vi "Validate Timing.vi"(8 "error in (no error)":errorcluster, 10 "Mode":T3="Standard-mode", 11 "I2C timing (ns)":T1 {"fSCL" format="%#_6p"}) -> (0 "error out":errorcluster, 1 "Timing violations":T2, 2 "Timing passed?":bool, 3 "I2C timing (ns) out":T1 {"fSCL" format="%#_6p"})   [LabVIEW 2009, in "IDW.lvlib"]
doc: "Validates timing parameters against contraints defined in the \"NXP UM10204, I2C-bus specification and user manual, Rev. 03\" document for most defined modes of operation.\n\nTiming constraints are provided for the following modes: Standard-mode (<b>Sm)</b>, Fast-mode (<b>Fm</b>), and Fast-mode Plus (<b>Fm+</b>)."
uses:
  IDW.lvlib
  _Typedefs/Bus mode.ctl
  _Typedefs/Timing - ns.ctl
  <vilib>/Utility/config.llb/Read Key (Double).vi
  <vilib>/Utility/config.llb/Read Key (I32).vi
  <vilib>/Utility/config.llb/NI_LVConfig.lvlib
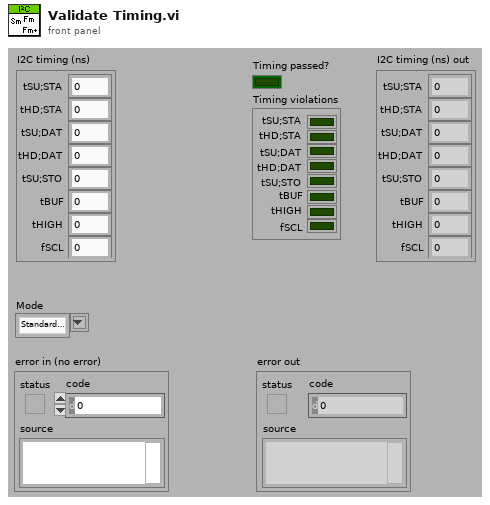
[diagram p1: front panel]
types:
  T1 = typedef "IDW.lvlib/Timing - ns.ctl" = cluster{"tSU;STA":i32, "tHD;STA":i32, "tSU;DAT":i32, "tHD;DAT":i32, "tSU;STO":i32, "tBUF":i32, "tHIGH":i32, "fSCL":dbl}
  T2 = cluster{"tSU;STA":bool, "tHD;STA":bool, "tSU;DAT":bool, "tHD;DAT":bool, "tSU;STO":bool, "tBUF":bool, "tHIGH":bool, "fSCL":bool}
  T3 = typedef "IDW.lvlib/Bus mode.ctl" = string
  T4 = typedef "NI_LVConfig.lvlib/Config Data RefNum.ctl" = refnum<k1>
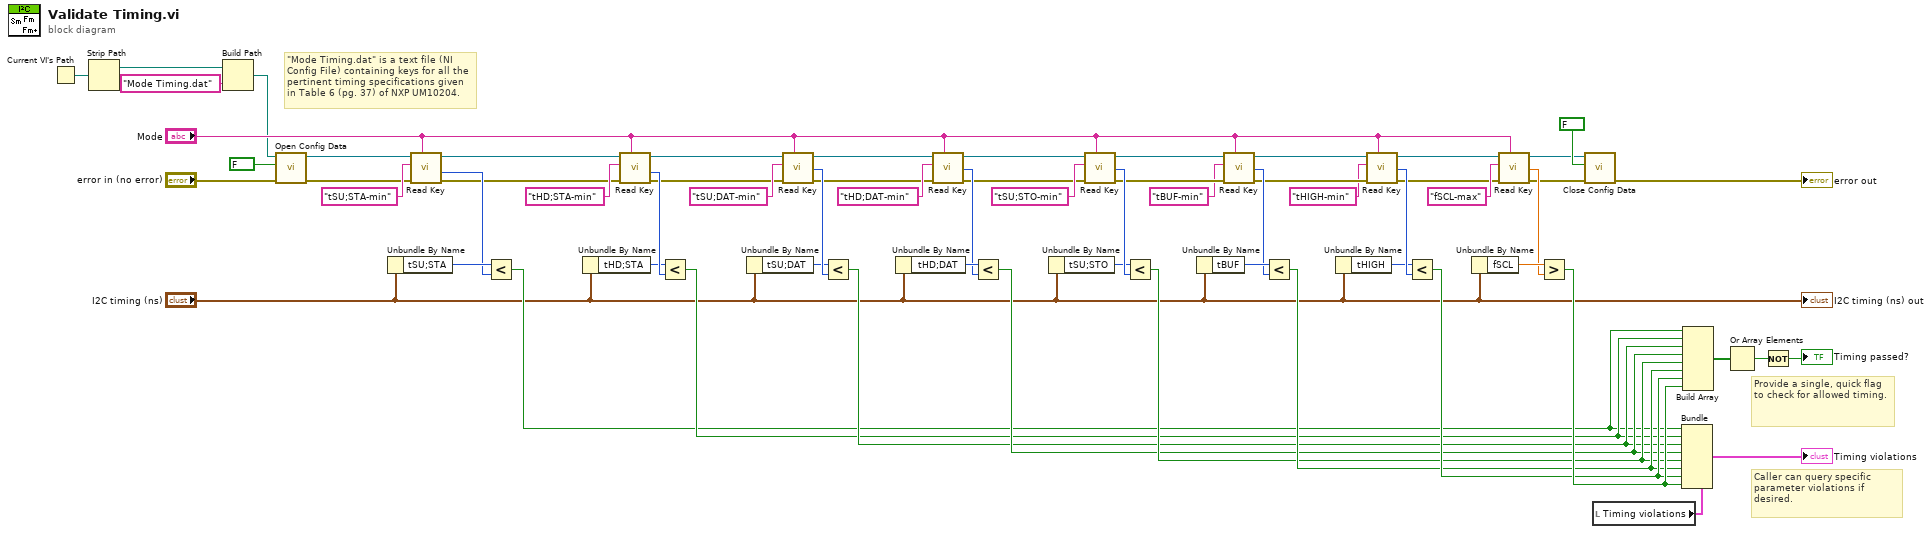
[diagram p0: block diagram]
diagram:
  # "Caller can query specific parameter violations if desired."
  # "Provide a single, quick flag to check for allowed timing."
  # "\"Mode Timing.dat\" is a text file (NI Config File) containing keys for all the pertinent timing specifications given in Table 6 (pg. 37) of NXP UM10204."
  n1 = Current VI's Path() -> (path=w65:path)
  n2 = Strip Path(path=w65) -> (stripped path=w64:path)  [unwired: 1 out]
  n3 = Build Path(base path=w64, name or relative path="Mode Timing.dat") -> (appended path=w2:path)
  n4 = call <vilib>:"Open Config Data.vi"("error in (no error)"="error in (no error)", "create file if necessary (T)"=FALSE ("create file if necessary? (T)"), "configuration file path"=w2) -> ("error out"=w4:errorcluster, "refnum"=w3:T4)  [unwired: 6 in, 1 out]
  n5 = Unbundle By Name("I2C timing (ns)") -> ("tSU;STA"=w60:i32)
  n6 = call-poly <vilib>:"Read Key.vi"("section"="Mode", "error in (no error)"=w4, "key"="tSU;STA-min", "refnum"=w3) -> ("error out"=w45:errorcluster, "value"=w59:i32, "refnum out"=w62:T4)  [unwired: 1 in, 4 out]
  n7 = Less?(x=w60, y=w59) -> (x < y?=w13:bool)
  n8 = Unbundle By Name("I2C timing (ns)") -> ("tHD;STA"=w56:i32)
  n9 = call-poly <vilib>:"Read Key.vi"("section"="Mode", "error in (no error)"=w45, "key"="tHD;STA-min", "refnum"=w62) -> ("error out"=w51:errorcluster, "value"=w57:i32, "refnum out"=w52:T4)  [unwired: 1 in, 4 out]
  n10 = Less?(x=w56, y=w57) -> (x < y?=w14:bool)
  n11 = Unbundle By Name("I2C timing (ns)") -> ("tSU;DAT"=w53:i32)
  n12 = call-poly <vilib>:"Read Key.vi"("section"="Mode", "error in (no error)"=w51, "key"="tSU;DAT-min", "refnum"=w52) -> ("error out"=w47:errorcluster, "value"=w54:i32, "refnum out"=w46:T4)  [unwired: 1 in, 4 out]
  n13 = Less?(x=w53, y=w54) -> (x < y?=w15:bool)
  n14 = Unbundle By Name("I2C timing (ns)") -> ("tHD;DAT"=w50:i32)
  n15 = call-poly <vilib>:"Read Key.vi"("section"="Mode", "error in (no error)"=w47, "key"="tHD;DAT-min", "refnum"=w46) -> ("error out"=w40:errorcluster, "value"=w49:i32, "refnum out"=w41:T4)  [unwired: 1 in, 4 out]
  n16 = Less?(x=w50, y=w49) -> (x < y?=w16:bool)
  n17 = Unbundle By Name("I2C timing (ns)") -> ("tSU;STO"=w42:i32)
  n18 = call-poly <vilib>:"Read Key.vi"("section"="Mode", "error in (no error)"=w40, "key"="tSU;STO-min", "refnum"=w41) -> ("error out"=w36:errorcluster, "value"=w43:i32, "refnum out"=w37:T4)  [unwired: 1 in, 4 out]
  n19 = Less?(x=w42, y=w43) -> (x < y?=w17:bool)
  n20 = Unbundle By Name("I2C timing (ns)") -> ("tBUF"=w39:i32)
  n21 = call-poly <vilib>:"Read Key.vi"("section"="Mode", "error in (no error)"=w36, "key"="tBUF-min", "refnum"=w37) -> ("error out"=w32:errorcluster, "value"=w38:i32, "refnum out"=w23:T4)  [unwired: 1 in, 4 out]
  n22 = Less?(x=w39, y=w38) -> (x < y?=w18:bool)
  n23 = Unbundle By Name("I2C timing (ns)") -> ("tHIGH"=w33:i32)
  n24 = call-poly <vilib>:"Read Key.vi"("section"="Mode", "error in (no error)"=w32, "key"="tHIGH-min", "refnum"=w23) -> ("error out"=w27:errorcluster, "value"=w34:i32, "refnum out"=w26:T4)  [unwired: 1 in, 4 out]
  n25 = Less?(x=w33, y=w34) -> (x < y?=w19:bool)
  n26 = Unbundle By Name("I2C timing (ns)") -> ("fSCL"=w29:dbl)
  n27 = call-poly <vilib>:"Read Key.vi"("section"="Mode", "error in (no error)"=w27, "key"="fSCL-max", "refnum"=w26) -> ("error out"=w8:errorcluster, "value"=w28:dbl, "refnum out"=w7:T4)  [unwired: 1 in, 4 out]
  n28 = Greater?(x=w29, y=w28) -> (0:w20:bool)
  n29 = call <vilib>:"Close Config Data.vi"("error in (no error)"=w8, "write file if changed (T)"=FALSE ("write configuration file? (T)"), "refnum"=w7) -> ("error out"=→"error out":errorcluster)  [unwired: 8 out]
  n30 = local read "Timing violations"() -> (w9:T2)
  n31 = Bundle(cluster=w9, "tSU;STA"=w13, "tHD;STA"=w14, "tSU;DAT"=w15, "tHD;DAT"=w16, "tSU;STO"=w17, "tBUF"=w18, "tHIGH"=w19, "fSCL"=w20) -> (→"Timing violations":T2)
  n32 = Build Array(w13, w14, w15, w16, w17, w18, w19, w20) -> (w12:bool[])
  n33 = Or Array Elements(Boolean array=w12) -> (logical OR=w11:bool)
  n34 = Not(x=w11) -> (.not. x?=→"Timing passed?":bool)
  "I2C timing (ns) out" <- "I2C timing (ns)"
